vi "BRig_Host_dataRunState__tSelectionPlot_get.vi"(7 "input_sSelection":u16, 8 "input_threshold_2":u16, 9 "input_threshold_1":u16, 11 "input_tSelection":u16) -> (3 "output_tSelection_plot":u16)   [LabVIEW 2014]
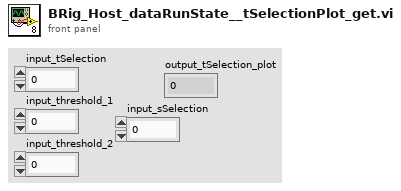
[diagram p1: front panel]
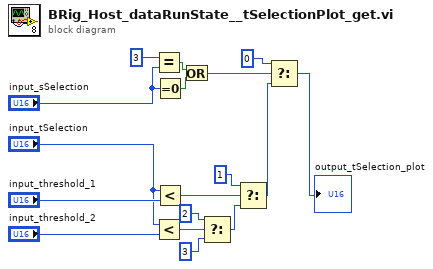
[diagram p0: block diagram]
diagram:
  n1 = Equal?(x=u16 3, y="input_sSelection") -> (x = y?=w7:bool)
  n2 = Less?(x="input_tSelection", y="input_threshold_2") -> (x < y?=w14:bool)
  n3 = Equal To 0?(x="input_sSelection") -> (x = 0?=w5:bool)
  n4 = Less?(x="input_tSelection", y="input_threshold_1") -> (x < y?=w10:bool)
  n5 = Or(x=w7, y=w5) -> (x .or. y?=w6:bool)
  n6 = Select(t=u16 2, s=w14, f=u16 3) -> (s? t:f=w11:u16)
  n7 = Select(t=u16 1, s=w10, f=w11) -> (s? t:f=w3:u16)
  n8 = Select(t=u16 0, s=w6, f=w3) -> (s? t:f=→"output_tSelection_plot":u16)
